vi "Over_Under_display.vi"(1 "Overflow array":dbl[][](array[numeric]) format="%.2f", 2 "Ch & spans":T2[](array[typedef])=[{"high limit (10V)"=10.0, "low limit (-10V)"=-10.0, "Ch No"=0, "Var name"="", "Use Latest Calib"=FALSE}, {"high limit (10V)"=10.0, "low limit (-10V)"=-10.0, "Ch No"=0, "Var name"="", "Use Latest Calib"=FALSE}, {"high limit (10V)"=10.0, "low limit (-10V)"=-10.0, "Ch No"=0, "Var name"="", "Use Latest Calib"=FALSE}] {"low limit (-10V)" format="%.3f"; "high limit (10V)" format="%.3f"}) -> (0 "Over/Under string":string)   [LabVIEW 2010]
uses:
  Controls/Ch_and_Spans.ctl
panel:
  out "Over/under array":T1(array[cluster]) {"% Underflows" format="%.5f"; "% Overflows" format="%.5f"}
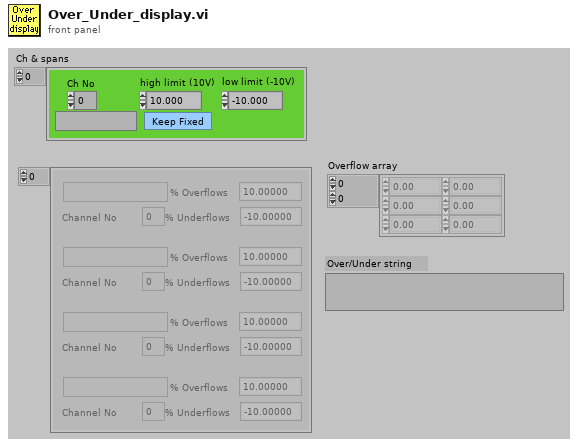
[diagram p1: front panel]
types:
  T1 = cluster{"% Overflows":dbl, "% Underflows":dbl, "Channel No":i16, "Var name":string}[]
  T2 = typedef "Ch_and_Spans.ctl" = cluster{"high limit (10V)":sgl, "low limit (-10V)":sgl, "Ch No":i16, "Var name":string, "Use Latest Calib":bool}
  T3 = cluster{"Overflows":dbl, "Underflows":dbl, "Channel No":i16, "Var name":string}
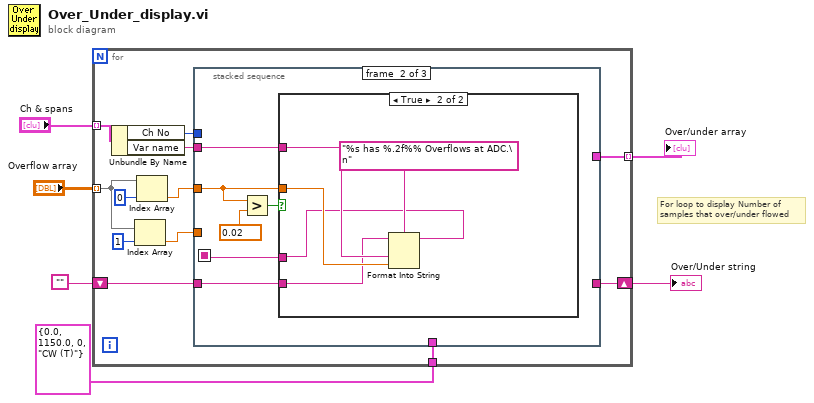
[diagram p0: block diagram]
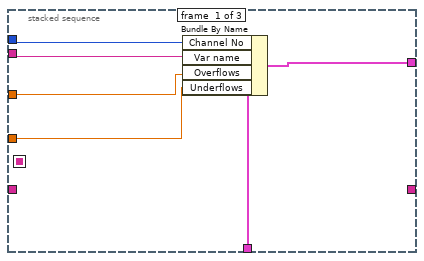
[diagram p2: hidden frame]
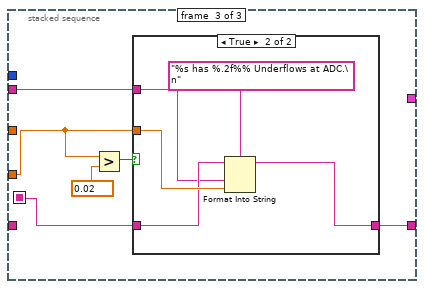
[diagram p4: hidden frame]
diagram:
  # "For loop to display Number of samples that over/under flowed"
  n1 = for {
    tunnel: "Ch & spans" -> [w18] mode=indexing
    tunnel: T3 {"Overflows"=0.0, "Underflows"=1150.0, "Channel No"=0, "Var name"="CW (T)"} -> [w17]
    tunnel: "Overflow array" -> [w16] mode=indexing
    tunnel: [w15] -> w4 mode=indexing
    shift-right: [w7] -> w2
    shift-left: "" -> [w8]
    n2 = Unbundle By Name(w18) -> ("Ch No"=w14:i16, "Var name"=w13:string)
    n3 = Index Array(array=w16, index=1) -> (element=w9:dbl)
    n4 = Index Array(array=w16, index=0) -> (element=w10:dbl)
    n5 = stacked-sequence {
      seq-local: [_ w28 _] -> [_ _ w41]
      tunnel: w9 -> [w24 _ w38]
      tunnel: w10 -> [w23 w27 _]
      tunnel: w13 -> [w22 w30 w42]
      tunnel: w14 -> [w21 _ _]
      tunnel: [w20 _ _] -> w15
      tunnel: w17 -> [w19 _ _]
      tunnel: w8 -> [_ w29 _]
      tunnel: [_ _ w40] -> w7
      frame #0 {
        n6 = Bundle By Name(cluster=w19, "Channel No"=w21, "Var name"=w22, "Overflows"=w23, "Underflows"=w24) -> (w20:T3)
      }
      frame #1 {
        n7 = Greater?(x=w27, y=0.02) -> (0:w25:bool)
        n8 = case shown="True" w25 {
          tunnel: w27 -> [_ w34]
          tunnel: w30 -> [_ w35]
          tunnel: w29 -> [w31 w33]
          tunnel: [w31 w32] -> w28
          frame False {
          }
          frame True {
            n9 = Format Into String(format string="%s has %.2f%% Overflows at ADC.\n" ("Format String"), initial string=w33, w35, w34) -> (resulting string=w32:string)  [unwired: 1 in, 1 out]
          }
        }
      }
      frame #2 {
        n10 = Greater?(x=w38, y=0.02) -> (0:w37:bool)
        n11 = case shown="True" w37 {
          tunnel: w38 -> [_ w48]
          tunnel: w42 -> [_ w44]
          tunnel: w41 -> [w43 w47]
          tunnel: [w43 w46] -> w40
          frame False {
          }
          frame True {
            n12 = Format Into String(format string="%s has %.2f%% Underflows at ADC.\n" ("Format String"), initial string=w47, w44, w48) -> (resulting string=w46:string)  [unwired: 1 in, 1 out]
          }
        }
      }
    }
  }
  "Over/under array" <- w4
  "Over/Under string" <- w2
